vi "center point.vi"(4 "border":cluster{dbl, dbl, dbl, dbl}) -> (1 "center":cluster{dbl, dbl})   [LabVIEW 2023]
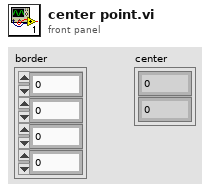
[diagram p1: front panel]
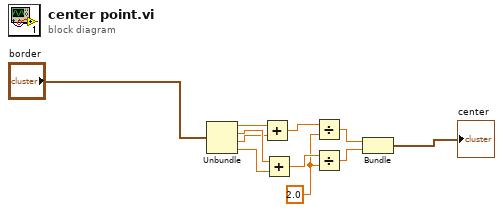
[diagram p0: block diagram]
diagram:
  w5 = 2.0 ("y")
  n1 = Unbundle("border") -> (w2:dbl, w6:dbl, w3:dbl, w7:dbl)
  n2 = Add(x=w2, y=w3) -> (x+y=w4:dbl)
  n3 = Add(x=w6, y=w7) -> (x+y=w8:dbl)
  n4 = Divide(x=w4, y=w5) -> (x/y=w10:dbl)
  n5 = Divide(x=w8, y=w5) -> (x/y=w9:dbl)
  n6 = Bundle(w10, w9) -> (→"center":cluster{dbl, dbl})  [unwired: 1 in]
